vi "PathPlanner_Path_NumPoints.vi"(11 "PathPlannerPath":T1={"Reversed"=FALSE, "RotationTargets"=[], "ConstraintZones"=[], "EventMarkers"=[], "GlobalConstraints"={"MaxVelocityMps;"=0.0, "MaxAccelerationMpsSq;"=0.0, "MaxAngularVelRadPsEc;"=0.0, "MaxAngularAccRadPSecSq"=0.0, "Exists"=FALSE, "Unlimited"=FALSE, "NominalVoltageVolts"=12.0}, "GoalEndState"={"VelocityMPS"=0.0, "Rotation"={"VALUE"=0.0, "COS"=1.0, "SIN"=0.0}}, "AllPoints"=[], "Name"="", "Waypoints"=[], "PointTowardsZones"=[], "IdealStartingState"={"VelocityMPS"=0.0, "Rotation"={"VALUE"=1.0, "COS"=0.0, "SIN"=0.0}}, "IsChoreoPath"=FALSE, "PreventFlipping"=FALSE} {"IdealStartingState"."Rotation"."SIN" format="%13.4f"; "IdealStartingState"."Rotation"."COS" format="%13.4f"; "IdealStartingState"."Rotation"."VALUE" format="%13.4f"; "PointTowardsZones"."TargetPosition"."Y" format="%14.3f"; "PointTowardsZones"."TargetPosition"."X" format="%14.3f"; "PointTowardsZones"."RotationOffset"."SIN" format="%13.4f"; "PointTowardsZones"."RotationOffset"."COS" format="%13.4f"; "PointTowardsZones"."RotationOffset"."VALUE" format="%13.4f"; "Waypoints"."nextControl"."Y" format="%14.3f"; "Waypoints"."nextControl"."X" format="%14.3f"; "Waypoints"."anchor"."Y" format="%14.3f"; "Waypoints"."anchor"."X" format="%14.3f"; "Waypoints"."prevControl"."Y" format="%14.3f"; "Waypoints"."prevControl"."X" format="%14.3f"; "AllPoints"."RotationTarget"."rotation"."SIN" format="%13.4f"; "AllPoints"."RotationTarget"."rotation"."COS" format="%13.4f"; "AllPoints"."RotationTarget"."rotation"."VALUE" format="%13.4f"; "AllPoints"."Position"."Y" format="%14.3f"; "AllPoints"."Position"."X" format="%14.3f"; "GoalEndState"."Rotation"."SIN" format="%13.4f"; "GoalEndState"."Rotation"."COS" format="%13.4f"; "GoalEndState"."Rotation"."VALUE" format="%13.4f"; "RotationTargets"."rotation"."SIN" format="%13.4f"; "RotationTargets"."rotation"."COS" format="%13.4f"; "RotationTargets"."rotation"."VALUE" format="%13.4f"}) -> (3 "NumPoints":i32)   [LabVIEW 2019, in "PathPlanner24.lvlib"]
doc: "Get the number of points in this path\n\nInputs: \n - Path - cluster - path definition data structure\n\nOutputs:\n - NumPoints - integer - Number of points in the path"
uses:
  PathPlanner24.lvlib
  <vilib>/Rock Robotics/WPI/ThirdParty/JAS_Junk/TrajLib/TypeDef/TRANSLATION2D.ctl
  <vilib>/Rock Robotics/WPI/ThirdParty/JAS_Junk/TrajLib/Trajectory_Library.lvlib
  <vilib>/Rock Robotics/WPI/ThirdParty/JAS_Junk/TrajLib/TypeDef/ROTATION2D.ctl
  TypeDef/PathPlannerPathConstraints.ctl
  TypeDef/PathPlannerRotationTarget.ctl
  TypeDef/PathPlannerConstraintsZone.ctl
  TypeDef/PathPlannerEventMarker.ctl
  TypeDef/PathPlannerGoalEndState.ctl
  TypeDef/PathPlannerPathPoint.ctl
  TypeDef/PathPlannerPath.ctl
  TypeDef/PathPlannerCommandUtil.ctl
  ENum/PathPlanner_TrajectoryEvent_Type_ENUM.ctl
  TypeDef/PathPlannerWaypoint.ctl
  TypeDef/PathPlannerPointTowardsZone.ctl
  TypeDef/PathPlannerIdealStartingState.ctl
  ENum/PathPlanner_CommandUtil_Type_ENUM.ctl
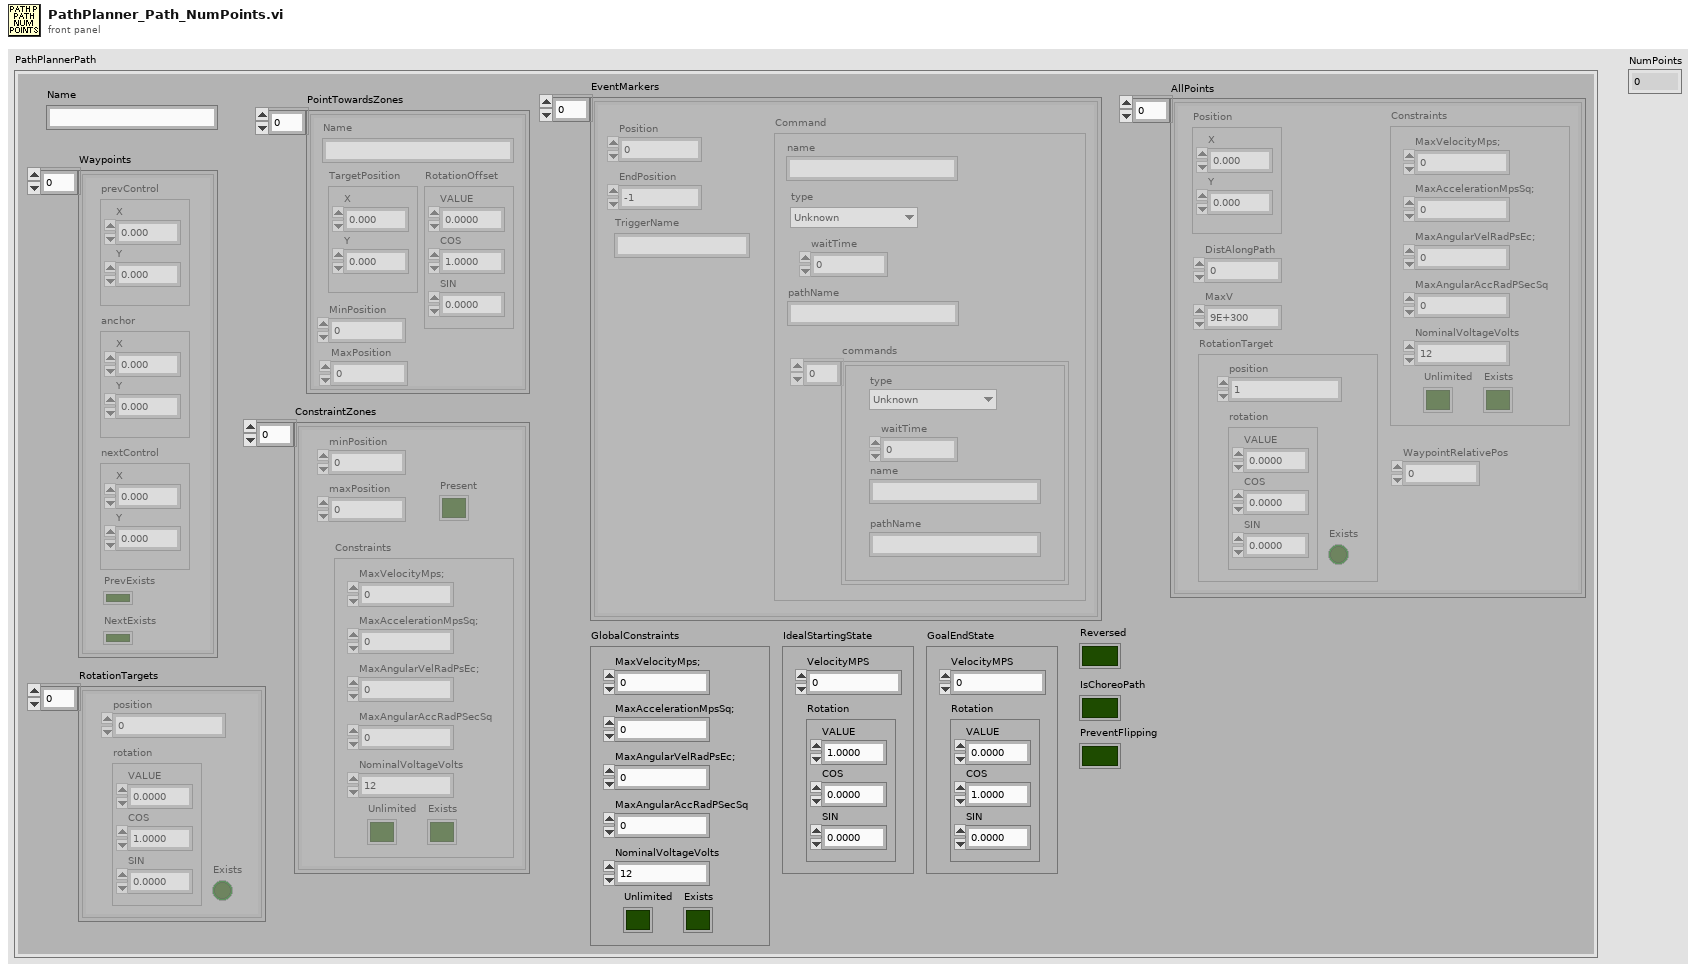
[diagram p1: front panel]
types:
  T1 = typedef "PathPlanner24.lvlib/PathPlannerPath.ctl" = cluster{"Reversed":bool, "RotationTargets":T2[], "ConstraintZones":T4[], "EventMarkers":T6[], "GlobalConstraints":T5, "GoalEndState":T10, "AllPoints":T11[], "Name":string, "Waypoints":T13[], "PointTowardsZones":T14[], "IdealStartingState":T15, "IsChoreoPath":bool, "PreventFlipping":bool}
  T2 = typedef "PathPlanner24.lvlib/PathPlannerRotationTarget.ctl" = cluster{"position":dbl, "rotation":T3, "Exists":bool}
  T3 = typedef "Trajectory_Library.lvlib/ROTATION2D.ctl" = cluster{"VALUE":dbl, "COS":dbl, "SIN":dbl}
  T4 = typedef "PathPlanner24.lvlib/PathPlannerConstraintsZone.ctl" = cluster{"minPosition":dbl, "maxPosition":dbl, "Constraints":T5, "Present":bool}
  T5 = typedef "PathPlanner24.lvlib/PathPlannerPathConstraints.ctl" = cluster{"MaxVelocityMps;":dbl, "MaxAccelerationMpsSq;":dbl, "MaxAngularVelRadPsEc;":dbl, "MaxAngularAccRadPSecSq":dbl, "Exists":bool, "Unlimited":bool, "NominalVoltageVolts":dbl}
  T6 = typedef "PathPlanner24.lvlib/PathPlannerEventMarker.ctl" = cluster{"Position":dbl, "Command":T7, "TriggerName":string, "EndPosition":dbl}
  T7 = typedef "PathPlanner24.lvlib/PathPlannerCommandUtil.ctl" = cluster{"waitTime":dbl, "name":string, "pathName":string, "commands":cluster{"type":T8, "waitTime":dbl, "name":string, "pathName":string}[], "type":T9}
  T8 = typedef "PathPlanner24.lvlib/PathPlanner_TrajectoryEvent_Type_ENUM.ctl" = enum16{"Unknown", "Wait", "Named", "Path", "Sequential", "Parallel", "Race", "Deadline", "PointTowardsZoneEnter", "PointTowardsZoneExit", "TriggerEventStart", "TriggerEventStop", "TriggerEventOneshot"}
  T9 = typedef "PathPlanner24.lvlib/PathPlanner_CommandUtil_Type_ENUM.ctl" = enum16{"Unknown", "Wait", "Named", "Path", "Sequential", "Parallel", "Race", "Deadline"}
  T10 = typedef "PathPlanner24.lvlib/PathPlannerGoalEndState.ctl" = cluster{"VelocityMPS":dbl, "Rotation":T3}
  T11 = typedef "PathPlanner24.lvlib/PathPlannerPathPoint.ctl" = cluster{"Position":T12, "DistAlongPath":dbl, "MaxV":dbl, "Constraints":T5, "RotationTarget":T2, "WaypointRelativePos":dbl}
  T12 = typedef "Trajectory_Library.lvlib/TRANSLATION2D.ctl" = cluster{"X":dbl, "Y":dbl}
  T13 = typedef "PathPlanner24.lvlib/PathPlannerWaypoint.ctl" = cluster{"prevControl":T12, "anchor":T12, "nextControl":T12, "PrevExists":bool, "NextExists":bool}
  T14 = typedef "PathPlanner24.lvlib/PathPlannerPointTowardsZone.ctl" = cluster{"RotationOffset":T3, "Name":string, "TargetPosition":T12, "MinPosition":dbl, "MaxPosition":dbl}
  T15 = typedef "PathPlanner24.lvlib/PathPlannerIdealStartingState.ctl" = cluster{"VelocityMPS":dbl, "Rotation":T3}
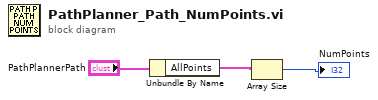
[diagram p0: block diagram]
diagram:
  n1 = Unbundle By Name("PathPlannerPath") -> ("AllPoints"=w2:T11[])
  n2 = Array Size(array=w2) -> (size(s)=→"NumPoints":i32)
